vi "PBar-Run Indeterminate.vi"() -> ()   [LabVIEW 2020]
panel:
  in  "Quit":bool
  in  "Slide":refnum<vi>
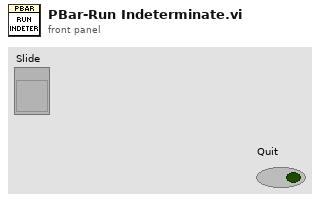
[diagram p1: front panel]
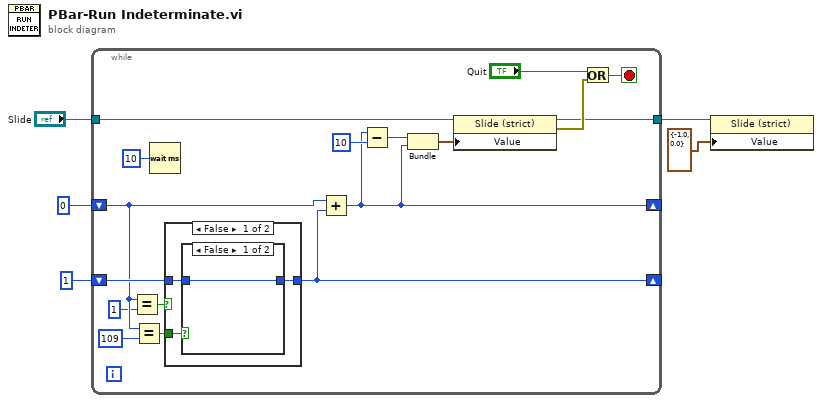
[diagram p0: block diagram]
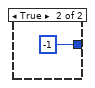
[diagram p2: hidden frame]
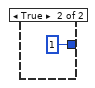
[diagram p3: hidden frame]
diagram:
  n1 = while {
    tunnel: "Slide" -> [w22]
    shift-right: [w17] -> _
    shift-left: 0 -> [w12]
    shift-right: [w15] -> _
    shift-left: 1 -> [w16]
    tunnel: [w6] -> w2
    stop <- w8 stop-if-true
    n2 = Equal?(x=w12, y=1) -> (x = y?=w10:bool)
    n3 = Equal?(x=w12, y=109) -> (x = y?=w13:bool)
    n4 = Wait (ms)(milliseconds to wait=u32 10) -> ()  [unwired: 1 out]
    n5 = case shown="False" w10 {
      tunnel: w16 -> [w23 _]
      tunnel: [w25 1 ("f")] -> w15
      tunnel: w13 -> [w24 _]
      frame False {
        n6 = case shown="False" w24 {
          tunnel: [w26 -1 ("f")] -> w25
          tunnel: w23 -> [w26 _]
          frame False {
          }
          frame True {
          }
        }
      }
      frame True {
      }
    }
    n7 = Add(x=w12, y=w15) -> (x+y=w17:i32)
    n8 = Subtract(x=w17, y=10) -> (x-y=w18:i32)
    n9 = Bundle(w18, w17) -> (w20:cluster{i32, i32})  [unwired: 1 in]
    n10 = property class="Slide (strict)"(reference=w22, "Value"=w20) -> (reference out=w6:refnum<vi>, error out=w7:errorcluster)  [unwired: 1 in]
    n11 = Or(x="Quit", y=w7) -> (x .or. y?=w8:bool)
  }
  n12 = property class="Slide (strict)"(reference=w2, "Value"=cluster{dbl, dbl} {-1.0, 0.0} ("Slide")) -> ()  [unwired: 1 in, 2 out]
